vi "Parse autobuild spec.vi"(8 "error in":errorcluster, 11 "Autobuild spec":path) -> (0 "error out":errorcluster, 3 "Tasks":T1[](array[typedef]), 5 "Retain Build":bool)   [LabVIEW 2013]
uses:
  Types/Task Info.ctl
  Types/Job Type.ctl
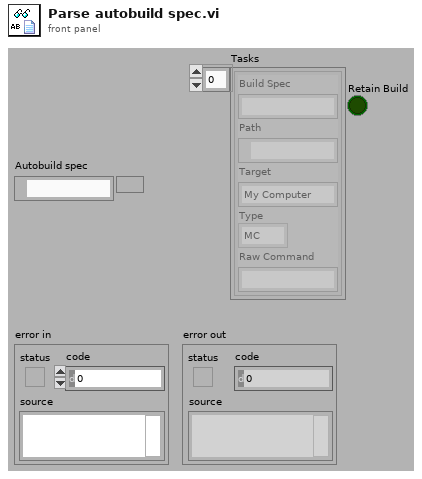
[diagram p1: front panel]
types:
  T1 = typedef "Task Info.ctl" = cluster{"Build Spec":string, "Path":path, "Target":string, "Type":T2, "Raw Command":string}
  T2 = typedef "Job Type.ctl" = enum16{"MC", "NOP", "VI", "Build", "VIP", "VIPB", "VIA"}
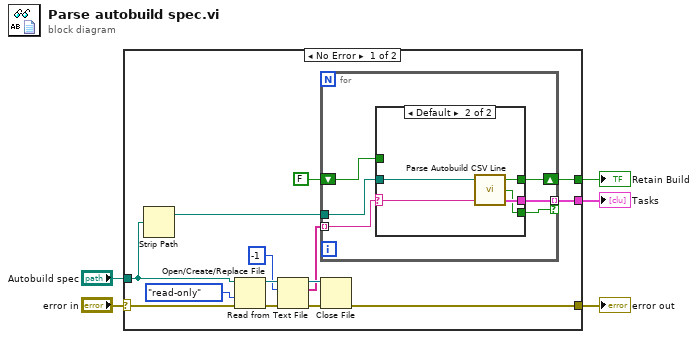
[diagram p0: block diagram]
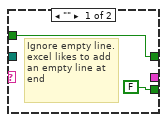
[diagram p2: hidden frame]
diagram:
  n1 = case shown="No Error" "error in" {
    selector: "error in" -> [w13 w33]
    tunnel: [w12 w33] -> w4
    tunnel: "Autobuild spec" -> [w10 _]
    tunnel: [w7 _] -> w2
    tunnel: [w6 _] -> w1
    frame No Error {
      n2 = Strip Path(path=w10) -> (stripped path=w9:path)  [unwired: 1 out]
      n3 = Open/Create/Replace File(file path (use dialog)=w10, error in=w13, access (0:read/write)=enum16{"read/write", "read-only", "write-only"}."read-only") -> (refnum out=w18:refnum<file>, error out=w17:errorcluster)  [unwired: 3 in, 1 out]
      n4 = Read from Text File(file (use dialog)=w18, count=-1, error in=w17) -> (refnum out=w15:refnum<file>, text=w11:string[], error out=w14:errorcluster)  [unwired: 1 in, 1 out]
      n5 = for {
        tunnel: w11 -> [w24] mode=indexing
        tunnel: w9 -> [w25]
        shift-right: [w21] -> w7
        shift-left: FALSE ("Retain Build") -> [w23]
        tunnel: [w22] -> w6 mode=indexing if=w20
        n6 = case shown="Default" w24 {
          selector: w24 -> [_ w30]
          tunnel: [_ w32] -> w22
          tunnel: w25 -> [_ w31]
          tunnel: [FALSE w29] -> w20
          tunnel: [w26 w28] -> w21
          tunnel: w23 -> [w26 _]
          frame "" {
            # "Ignore empty line. excel likes to add an empty line at end"
          }
          frame Default {
            n7 = call "Parse Autobuild CSV Line.vi"("String"=w30, "Autobuild root dir"=w31) -> ("Task Info"=w32:T1, "Build Command"=w29:bool, "Retain Build"=w28:bool)  [unwired: 1 in]
          }
        }
      }
      n8 = Close File(refnum=w15, error in=w14) -> (error out=w12:errorcluster)  [unwired: 1 out]
    }
    frame Error {
    }
  }
  "error out" <- w4
  "Tasks" <- w1
  "Retain Build" <- w2
